vi "Lower Compress Stop.vi"(8 "error in (no error)":errorcluster, 9 "Gantry In":refnum<k24>, 10 "I-O.lvclass":refnum<class "I-O.lvclass">, 11 "Pick and Place in":refnum<class "Pick and Place.lvclass">) -> (0 "error out":errorcluster, 1 "Gantry Out":refnum<k24>, 2 "I-O out":refnum<class "I-O.lvclass">, 3 "Pick and Place Out":refnum<class "Pick and Place.lvclass">)   [LabVIEW 2020, in "Pick and Place.lvclass"]
uses:
  Pick and Place.lvclass
  Controller/I-O/I-O.lvclass
  Drivers/Aerotech A3200/Aerotech.lvlib
  Controller/Motion/A3200/A3200.lvclass
  C:/Program Files (x86)/Aerotech/A3200/LabVIEW/2010/Bin/Aerotech.A3200.dll
  Program Files (x86)/Aerotech/A3200/LabVIEW/2010/Bin/Aerotech.A3200.dll
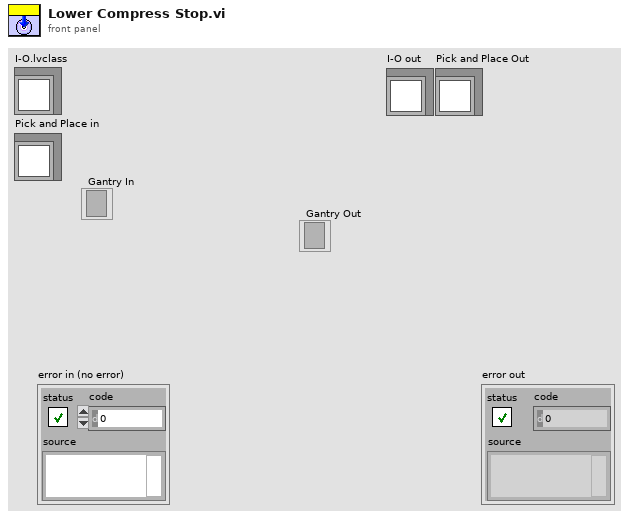
[diagram p1: front panel]
types:
  T1 = typedef "I-O.lvclass/Pin Map.ctl" = cluster{"Region Valves":i32[], "Extra Valves":dbl[][][], "Tool Primary Valve":i32, "Tool Secondary Valve":i32, "Region Sensors":i32[], "Extra Sensors":dbl[][][], "Tool Primary Sensor":dbl, "Tool Secondary Sensor":dbl, "Compression Sensor":dbl, "5V":i32, "Dispenser Sensor":dbl}
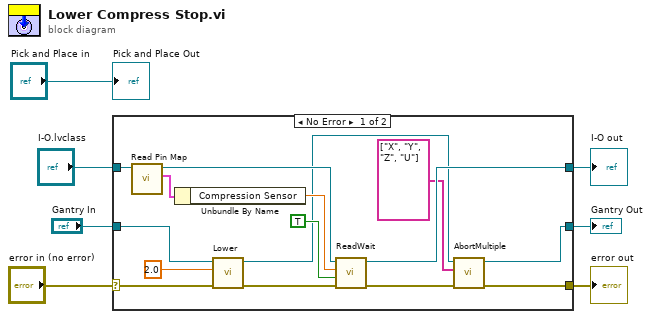
[diagram p0: block diagram]
diagram:
  n1 = case shown="No Error" "error in (no error)" {
    selector: "error in (no error)" -> [w9 w25]
    tunnel: [w8 w25] -> w6
    tunnel: "I-O.lvclass" -> [w20 w24]
    tunnel: [w22 w24] -> w4
    tunnel: "Gantry In" -> [w16 w23]
    tunnel: [w11 w23] -> w1
    frame No Error {
      n2 = call-dynamic "Read Pin Map.vi"("I-O in"=w20) -> ("Pin Map 2"=w18:T1, "I-O out"=w19:refnum<class "I-O.lvclass">)  [unwired: 8 in, 1 out]
      n3 = Unbundle By Name(w18) -> ("Compression Sensor"=w21:dbl)
      n4 = call "Lower.vi"("error in (no error)"=w9, "Speed"=2.0, "Gantry In"=w16) -> ("error out"=w14:errorcluster, "Gantry Out"=w13:refnum<k24>)  [unwired: 7 in]
      n5 = call "ReadWait.vi"("error in (no error)"=w14, "Value"=TRUE, "Read"=w21, "I-O in"=w19) -> ("error out"=w10:errorcluster, "I-O out"=w22:refnum<class "I-O.lvclass">)  [unwired: 6 in]
      n6 = call "AbortMultiple.vi"("error in (no error)"=w10, "axis names"=string[] ["X", "Y", "Z", "U"], "controller in"=w13) -> ("error out"=w8:errorcluster, "controller out"=w11:refnum<k24>)  [unwired: 7 in]
    }
    frame Error {
    }
  }
  "error out" <- w6
  "I-O out" <- w4
  "Gantry Out" <- w1
  "Pick and Place Out" <- "Pick and Place in"
